vi "1_ImClass(Train).vi"() -> ()   [LabVIEW 2020]
doc: "This example demonstrates the usage of Deep Learning Toolkit for solving hand written digit recognition problem with Convolutional Neural Network (CNN).\n\nDataset: MNIST http://yann.lecun.com/exdb/mnist/\nRequirements: Deep Learning Toolkit for LabVIEW."
uses:
  <vilib>/Ngene/Deep Learning Toolkit/Toolkit/NN_Train/Controls/NN_Train_Params.ctl
  <vilib>/Ngene/Deep Learning Toolkit/Toolkit/NN_Train/Controls/NN_Train_Optimizer.ctl
  <vilib>/Ngene/Deep Learning Toolkit/Toolkit/NN_Train/Controls/NN_Train_Data_Sampling.ctl
  Controls/Img_RGB.ctl
  <vilib>/Ngene/Deep Learning Toolkit/Toolkit/NN_Train/Controls/NN_Train_Session_Data.ctl
  <vilib>/Ngene/Deep Learning Toolkit/Toolkit/NN_Train/Controls/NN_LR_Policy_Cfg.ctl
  <vilib>/Ngene/Deep Learning Toolkit/Toolkit/NN_Train/Controls/NN_LR_Policy_Type.ctl
  <vilib>/Ngene/Deep Learning Toolkit/Toolkit/NN_Network/Controls/NN_Device.ctl
  <vilib>/Ngene/Deep Learning Toolkit/Toolkit/NN_Layers/Layers/FC/Controls/NN_Layer_Config(FC).ctl
  <vilib>/Ngene/Deep Learning Toolkit/Toolkit/NN_Layers/Layers/BatchNorm/Controls/NN_BN_Params.ctl
  <vilib>/Ngene/Deep Learning Toolkit/Toolkit/NN_Activations/Controls/NN_Activation_Type.ctl
  <vilib>/Ngene/Deep Learning Toolkit/Toolkit/NN_Layers/Controls/NN_Layer_Init_Params.ctl
  <vilib>/Ngene/Deep Learning Toolkit/Toolkit/NN_Layers/Controls/NN_Layer_Weight_Init_Type.ctl
  <vilib>/Ngene/Deep Learning Toolkit/Toolkit/NN_Layers/Layers/Input/Controls/NN_Layer_Config(Input3D).ctl
  <vilib>/Ngene/Deep Learning Toolkit/Toolkit/NN_Data/API/NN_Dims(C,H,W).ctl
  <vilib>/Ngene/Deep Learning Toolkit/Toolkit/NN_Data/Controls/NN_Data_type.ctl
  <vilib>/Ngene/Deep Learning Toolkit/Toolkit/NN_Network/Controls/NN_Save_Before_Destroy_Options.ctl
  <vilib>/Ngene/Deep Learning Toolkit/Toolkit/NN_Layers/Layers/Input/Controls/NN_Layer_Config_Aug(Input3D).ctl
  <vilib>/Ngene/Deep Learning Toolkit/Toolkit/NN_Layers/Layers/Input/Controls/Aug/NN_Input3D_Aug_Config.ctl
  <vilib>/Ngene/Deep Learning Toolkit/Toolkit/NN_Layers/Layers/Input/Controls/Aug/NN_Input3D_Aug_Types.ctl
  <vilib>/Ngene/Deep Learning Toolkit/Toolkit/NN_Layers/Layers/Input/Controls/Aug/Aug_Distribution_Type.ctl
  <vilib>/Ngene/Deep Learning Toolkit/Toolkit/NN_Layers/Layers/Input/NN_Layer_Create(Input3D).vi
  <vilib>/Ngene/Deep Learning Toolkit/Toolkit/NN_Layers/Layers/FC/NN_Layer_Create(FC).vi
  <vilib>/Ngene/Deep Learning Toolkit/Toolkit/NN_Layers/Layers/SoftMax/NN_Layer_Create(SoftMax).vi
  <vilib>/Ngene/Deep Learning Toolkit/Toolkit/NN_Train/Loss_Functions/NN_Set_Loss(CrossEntropy).vi
  <vilib>/Ngene/Deep Learning Toolkit/Toolkit/NN_Network/subVIs/NN_Predict/NN_Predict(In3D_Out1D).vi
  <vilib>/Ngene/Deep Learning Toolkit/Toolkit/NN_Train/Eval_Loss/NN_Eval_Test_Error_Loss/NN_Eval(In3D_Out1D).vi
  <vilib>/Ngene/Deep Learning Toolkit/Toolkit/NN_Train/Eval_Loss/NN_Calc_Cofusion_Matrix/NN_Calc_Confusion_Matrix(In3D_Out1D).vi
  <vilib>/Ngene/Deep Learning Toolkit/Toolkit/NN_Data/subVIs/Dataset_Destroy/NN_Datasets_All_Destroy(In3D_Out1D).vi
  <vilib>/Ngene/Deep Learning Toolkit/Toolkit/Deep_Learning_Toolkit_by_Ngene.lvlib
  <vilib>/ptbypt/NI_PtbyPt.lvlib
panel:
  in  "Tab":T1(tab)
  out "Train/Val_Metrics":T2={"Train_Loss"=0.32149845391511916, "Test_Loss"=0.4582325220108032, "Test_Error"=0.14990000426769257} {"Test_Error" format="%#_4g"; "Test_Loss" format="%#_4g"; "Train_Loss" format="%#_4g"}
  in  "Test Images":path=path "D:/DNN/CIFAR-10_Images/Test"
  out "Train Speed (s/iter)":dbl=2166.5318226281724 format="%#_3p"
  out "Train Graphs":T3(graph)={"mean"=0.32149845391511916, "Valid_Loss"=0.45823252, "Valid_Error"=0.1499}
  in  "Eval Test":bool
  out "Session Data":T4={"Epochs"=22.9248, "Tot_Iter"=8955, "LR"=1.25e-05, "LR_iter"=8956}
  in  "Stop":bool
  in  "LR Update Policy":T5={"Policy_Type"=enum."Step", "LR0"=0.0002, "k"=5.0, "WarmUp_Policy"=enum."Step", "WarmUp_Iter"=100, "WarmUp_Ratio"=100.0} {"WarmUp_Ratio" min=1; "WarmUp_Iter" min=1; "LR0" format="%.7f"}
  out "Train Speed (s/iter)":dbl=0.05908060000001569 format="%#_2p"
  in  "Train_Params":T7={"Optimizer"=enum."Adam", "Beta_1"=0.9, "Beta_2"=0.999, "Weight Decay(L1)"=1e-07, "Weight Decay(L2)"=1e-07, "Data_Sampling"=enum."Random"}
  out "Time_Elapsed":dbl=534.0725416999994 format="%<%H:%M:%S>t"
  in  "Working Dir":path=path "D:/working"
  in  "Train Images":path=path "D:/DNN/CIFAR-10_Images/Train"
  in  "NN_Device":T10=enum."GPU"
  out "Incorrectly Classified Imgs":T11[][](array[typedef])=[[{"image"=bytes[30030], "Truth"="airplane", "Predicted"="truck", "Name"="airplane_00003.bmp"}, {"image"=bytes[30030], "Truth"="airplane", "Predicted"="ship", "Name"="airplane_00052.bmp"}, {"image"=bytes[30030], "Truth"="airplane", "Predicted"="bird", "Name"="airplane_00125.bmp"}, {"image"=bytes[30030], "Truth"="airplane", "Predicted"="ship", "Name"="airplane_00169.bmp"}, {"image"=bytes[30030], "Truth"="airplane", "Predicted"="cat", "Name"="airplane_00180.bmp"}, {"image"=bytes[30030], "Truth"="airplane", "Predicted"="truck", "Name"="airplane_00237.bmp"}, {"image"=bytes[30030], "Truth"="airplane", "Predicted"="deer", "Name"="airplane_00255.bmp"}, {"image"=bytes[30030], "Truth"="airplane", "Predicted"="ship", "Name"="airplane_00264.bmp"}, {"image"=bytes[30030], "Truth"="airplane", "Predicted"="automobile", "Name"="airplane_00281.bmp"}, {"image"=bytes[30030], "Truth"="airplane", "Predicted"="truck", "Name"="airplane_00284.bmp"}], [{"image"=bytes[30030], "Truth"="airplane", "Predicted"="ship", "Name"="airplane_00287.bmp"}, {"image"=bytes[30030], "Truth"="airplane", "Predicted"="bird", "Name"="airplane_00313.bmp"}, {"image"=bytes[30030], "Truth"="airplane", "Predicted"="ship", "Name"="airplane_00376.bmp"}, {"image"=bytes[30030], "Truth"="airplane", "Predicted"="bird", "Name"="airplane_00378.bmp"}, {"image"=bytes[30030], "Truth"="airplane", "Predicted"="truck", "Name"="airplane_00398.bmp"}, {"image"=bytes[30030], "Truth"="airplane", "Predicted"="frog", "Name"="airplane_00428.bmp"}, {"image"=bytes[30030], "Truth"="airplane", "Predicted"="truck", "Name"="airplane_00473.bmp"}, {"image"=bytes[30030], "Truth"="airplane", "Predicted"="ship", "Name"="airplane_00477.bmp"}, {"image"=bytes[30030], "Truth"="airplane", "Predicted"="bird", "Name"="airplane_00491.bmp"}, {"image"=bytes[30030], "Truth"="airplane", "Predicted"="ship", "Name"="airplane_00526.bmp"}], [{"image"=bytes[30030], "Truth"="airplane", "Predicted"="cat", "Name"="airplane_00531.bmp"}, {"image"=bytes[30030], "Truth"="airplane", "Predicted"="ship", "Name"="airplane_00581.bmp"}, {"image"=bytes[30030], "Truth"="airplane", "Predicted"="automobile", "Name"="airplane_00675.bmp"}, {"image"=bytes[30030], "Truth"="airplane", "Predicted"="bird", "Name"="airplane_00678.bmp"}, {"image"=bytes[30030], "Truth"="airplane", "Predicted"="cat", "Name"="airplane_00689.bmp"}, {"image"=bytes[30030], "Truth"="airplane", "Predicted"="truck", "Name"="airplane_00767.bmp"}, {"image"=bytes[30030], "Truth"="airplane", "Predicted"="automobile", "Name"="airplane_00814.bmp"}, {"image"=bytes[30030], "Truth"="airplane", "Predicted"="truck", "Name"="airplane_00822.bmp"}, {"image"=bytes[30030], "Truth"="airplane", "Predicted"="ship", "Name"="airplane_00841.bmp"}, {"image"=bytes[30030], "Truth"="airplane", "Predicted"="ship", "Name"="airplane_00885.bmp"}], [{"image"=bytes[30030], "Truth"="airplane", "Predicted"="truck", "Name"="airplane_00886.bmp"}, {"image"=bytes[30030], "Truth"="airplane", "Predicted"="ship", "Name"="airplane_00888.bmp"}, {"image"=bytes[30030], "Truth"="airplane", "Predicted"="cat", "Name"="airplane_00912.bmp"}, {"image"=bytes[30030], "Truth"="airplane", "Predicted"="dog", "Name"="airplane_00982.bmp"}, {"image"=bytes[30030], "Truth"="airplane", "Predicted"="ship", "Name"="airplane_01001.bmp"}, {"image"=bytes[30030], "Truth"="airplane", "Predicted"="automobile", "Name"="airplane_01072.bmp"}, {"image"=bytes[30030], "Truth"="airplane", "Predicted"="ship", "Name"="airplane_01090.bmp"}, {"image"=bytes[30030], "Truth"="airplane", "Predicted"="ship", "Name"="airplane_01093.bmp"}, {"image"=bytes[30030], "Truth"="airplane", "Predicted"="automobile", "Name"="airplane_01109.bmp"}, {"image"=bytes[30030], "Truth"="airplane", "Predicted"="ship", "Name"="airplane_01137.bmp"}], [{"image"=bytes[30030], "Truth"="airplane", "Predicted"="truck", "Name"="airplane_01241.bmp"}, {"image"=bytes[30030], "Truth"="airplane", "Predicted"="truck", "Name"="airplane_01322.bmp"}, {"image"=bytes[30030], "Truth"="airplane", "Predicted"="truck", "Name"="airplane_01461.bmp"}, {"image"=bytes[30030], "Truth"="airplane", "Predicted"="ship", "Name"="airplane_01463.bmp"}, {"image"=bytes[30030], "Truth"="airplane", "Predicted"="truck", "Name"="airplane_01514.bmp"}, {"image"=bytes[30030], "Truth"="airplane", "Predicted"="ship", "Name"="airplane_01574.bmp"}, {"image"=bytes[30030], "Truth"="airplane", "Predicted"="bird", "Name"="airplane_01714.bmp"}, {"image"=bytes[30030], "Truth"="airplane", "Predicted"="ship", "Name"="airplane_01718.bmp"}, {"image"=bytes[30030], "Truth"="airplane", "Predicted"="ship", "Name"="airplane_01739.bmp"}, {"image"=bytes[30030], "Truth"="airplane", "Predicted"="bird", "Name"="airplane_01785.bmp"}], [{"image"=bytes[30030], "Truth"="airplane", "Predicted"="ship", "Name"="airplane_01796.bmp"}, {"image"=bytes[30030], "Truth"="airplane", "Predicted"="horse", "Name"="airplane_01823.bmp"}, {"image"=bytes[30030], "Truth"="airplane", "Predicted"="cat", "Name"="airplane_01898.bmp"}, {"image"=bytes[30030], "Truth"="airplane", "Predicted"="ship", "Name"="airplane_01926.bmp"}, {"image"=bytes[30030], "Truth"="airplane", "Predicted"="automobile", "Name"="airplane_02085.bmp"}, {"image"=bytes[30030], "Truth"="airplane", "Predicted"="bird", "Name"="airplane_02091.bmp"}, {"image"=bytes[30030], "Truth"="airplane", "Predicted"="truck", "Name"="airplane_02136.bmp"}, {"image"=bytes[30030], "Truth"="airplane", "Predicted"="cat", "Name"="airplane_02232.bmp"}, {"image"=bytes[30030], "Truth"="airplane", "Predicted"="ship", "Name"="airplane_02248.bmp"}, {"image"=bytes[30030], "Truth"="airplane", "Predicted"="automobile", "Name"="airplane_02276.bmp"}], [{"image"=bytes[30030], "Truth"="airplane", "Predicted"="bird", "Name"="airplane_02322.bmp"}, {"image"=bytes[30030], "Truth"="airplane", "Predicted"="ship", "Name"="airplane_02379.bmp"}, {"image"=bytes[30030], "Truth"="airplane", "Predicted"="deer", "Name"="airplane_02404.bmp"}, {"image"=bytes[30030], "Truth"="airplane", "Predicted"="ship", "Name"="airplane_02473.bmp"}, {"image"=bytes[30030], "Truth"="airplane", "Predicted"="automobile", "Name"="airplane_02490.bmp"}, {"image"=bytes[30030], "Truth"="airplane", "Predicted"="automobile", "Name"="airplane_02532.bmp"}, {"image"=bytes[30030], "Truth"="airplane", "Predicted"="bird", "Name"="airplane_02548.bmp"}, {"image"=bytes[30030], "Truth"="airplane", "Predicted"="truck", "Name"="airplane_02587.bmp"}, {"image"=bytes[30030], "Truth"="airplane", "Predicted"="bird", "Name"="airplane_02622.bmp"}, {"image"=bytes[30030], "Truth"="airplane", "Predicted"="ship", "Name"="airplane_02672.bmp"}], [{"image"=bytes[30030], "Truth"="airplane", "Predicted"="ship", "Name"="airplane_02704.bmp"}, {"image"=bytes[30030], "Truth"="airplane", "Predicted"="automobile", "Name"="airplane_02782.bmp"}, {"image"=bytes[30030], "Truth"="airplane", "Predicted"="ship", "Name"="airplane_02958.bmp"}, {"image"=bytes[30030], "Truth"="airplane", "Predicted"="bird", "Name"="airplane_02968.bmp"}, {"image"=bytes[30030], "Truth"="airplane", "Predicted"="truck", "Name"="airplane_02976.bmp"}, {"image"=bytes[30030], "Truth"="airplane", "Predicted"="cat", "Name"="airplane_03097.bmp"}, {"image"=bytes[30030], "Truth"="airplane", "Predicted"="bird", "Name"="airplane_03100.bmp"}, {"image"=bytes[30030], "Truth"="airplane", "Predicted"="ship", "Name"="airplane_03158.bmp"}, {"image"=bytes[30030], "Truth"="airplane", "Predicted"="bird", "Name"="airplane_03164.bmp"}, {"image"=bytes[30030], "Truth"="airplane", "Predicted"="automobile", "Name"="airplane_03171.bmp"}]]
  out "Confusion Matrix":string[][](table)=[["771", "28", "44", "15", "13", "3", "5", "5", "71", "45", "0.7710"], ["6", "928", "0", "2", "3", "1", "1", "1", "10", "48", "0.9280"], ["35", "4", "727", "51", "62", "48", "34", "12", "21", "6", "0.7270"], ["15", "6", "46", "665", "29", "149", "33", "16", "22", "19", "0.6650"], ["2", "1", "47", "57", "800", "35", "12", "32", "12", "2", "0.8000"], ["2", "1", "32", "134", "13", "768", "12", "22", "6", "10", "0.7680"], ["5", "4", "42", "66", "34", "15", "822", "3", "6", "3", "0.8220"], ["5", "1", "15", "64", "51", "67", "4", "781", "2", "10", "0.7810"], ["33", "23", "3", "3", "2", "1", "1", "0", "905", "29", "0.9050"], ["4", "37", "4", "4", "1", "2", "2", "1", "16", "929", "0.9290"], ["0.8781", "0.8984", "0.7573", "0.6268", "0.7937", "0.7052", "0.8877", "0.8946", "0.8450", "0.8438", ""]]
  out "Test_Error(Final)":sgl=0.1904
  out "Test_Loss(Final)":sgl=0.544509 format="%#_3g"
  out "Test_Error":sgl=0.1945
  out "Test_Loss":sgl=0.57450217
  # "6. Periodically press \"Eval Test\" button to evaluate Test Loss/Error.\n7. Hit the \"Stop\" button when the Test loss/errors stops decreasing.\n8. Go to the \"Incorrectly Classified Images\" tab to view images from the test dataset that were incorrectly classified.\n9. Navigate to the \"Confusion Matrix\" tab to analyze the classification performance across all classes.\n10. Check the files generated in the \"Working Dir\" directory. A subdirectory with the network name will be created, containing three files: the model configuration file (.cfg), trained weights file (.bin), and a network visualization file (.svg) that can be opened in a web browser.\n\nMore Examples:  https://github.com/ngenehub/deepltk_examples"
  # "Overview: This example demonstrates the usage of Deep Learning Toolkit for solving image classification problem.\nRequirements: \nDeep Learning Toolkit for LabVIEW.\nNI Vision Development Module.\nInstructions:\n1. Provide the train and test dataset paths in the \"Train Images\" and \"Test Images\" control .\n2. Set appropriate path at \"Working Dir\" control where the results of the training will be stored.\n3. Select CPU or GPU at \"NN_Device\" depending on GPU availability.\n4. Run the VI with current configuration of the training parameters and Learning Rate update policy.\n5. Observe how the training loss is decreasing."
  # "Displaying images from the dataset that were incorrectly classified by the trained network."
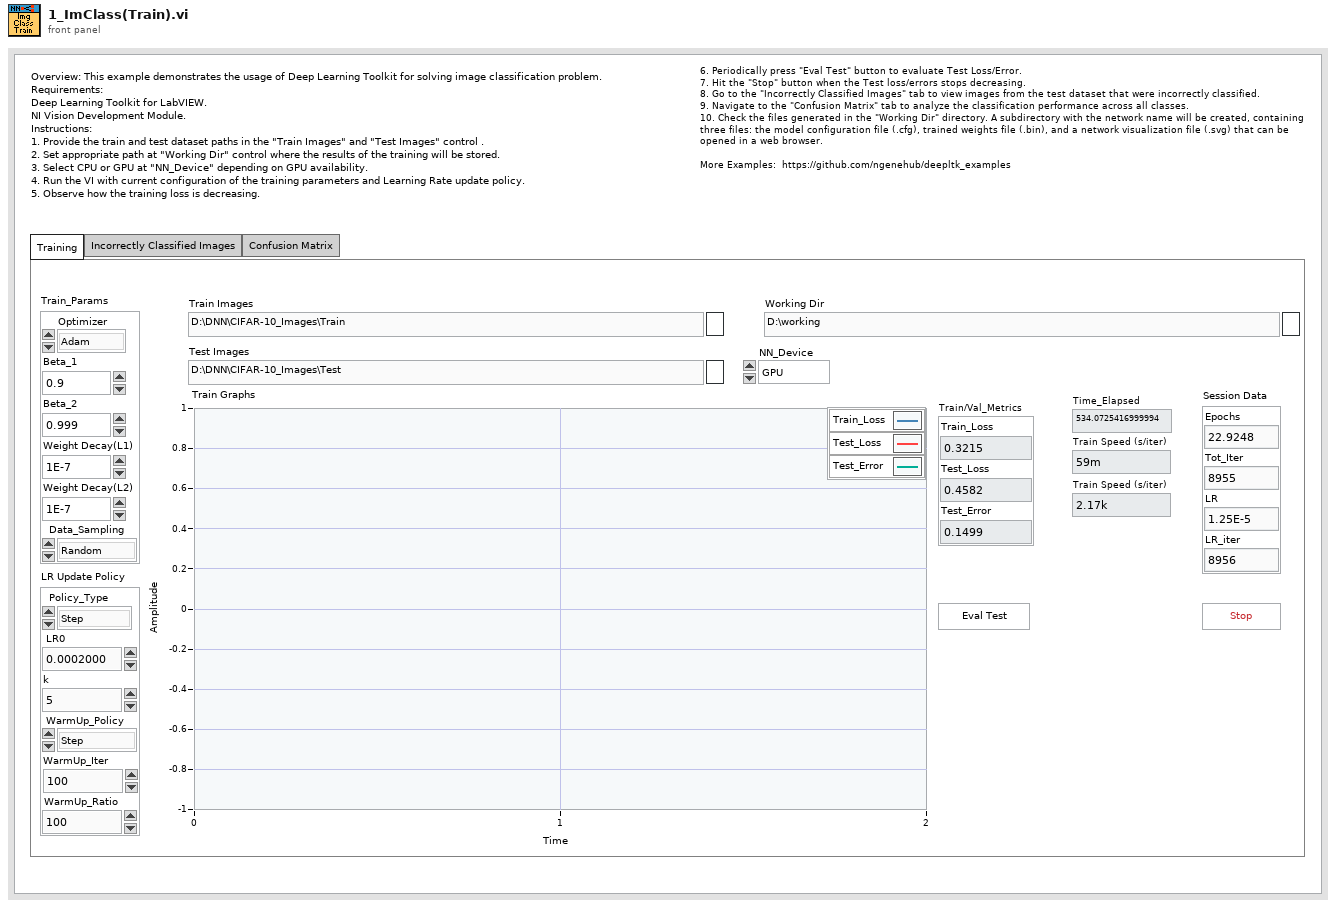
[diagram p1: front panel]
types:
  T1 = enum32{"Training", "Incorrectly Classified Images", "Confusion Matrix"}
  T2 = cluster{"Train_Loss":dbl, "Test_Loss":dbl, "Test_Error":dbl}
  T3 = cluster{"mean":dbl, "Valid_Loss":sgl, "Valid_Error":sgl}
  T4 = typedef "Deep_Learning_Toolkit_by_Ngene.lvlib/NN_Train_Session_Data.ctl" = cluster{"Epochs":sgl, "Tot_Iter":i32, "LR":sgl, "LR_iter":i32}
  T5 = typedef "Deep_Learning_Toolkit_by_Ngene.lvlib/NN_LR_Policy_Cfg.ctl" = cluster{"Policy_Type":T6, "LR0":dbl, "k":sgl, "WarmUp_Policy":enum16{"Step", "Ramp"}, "WarmUp_Iter":i32, "WarmUp_Ratio":sgl}
  T6 = typedef "Deep_Learning_Toolkit_by_Ngene.lvlib/NN_LR_Policy_Type.ctl" = enum16{"Manual", "Step", "Exp", "1/t"}
  T7 = typedef "Deep_Learning_Toolkit_by_Ngene.lvlib/NN_Train_Params.ctl" = cluster{"Optimizer":T8, "Beta_1":sgl, "Beta_2":sgl, "Weight Decay(L1)":sgl, "Weight Decay(L2)":sgl, "Data_Sampling":T9}
  T8 = typedef "Deep_Learning_Toolkit_by_Ngene.lvlib/NN_Train_Optimizer.ctl" = enum16{"SGD", "Adam", "Adagrad", "Adadelta", "RMSProp", "Nesterov"}
  T9 = typedef "Deep_Learning_Toolkit_by_Ngene.lvlib/NN_Train_Data_Sampling.ctl" = enum16{"Random", "Sequential"}
  T10 = typedef "Deep_Learning_Toolkit_by_Ngene.lvlib/NN_Device.ctl" = enum16{"CPU", "GPU"}
  T11 = typedef "Img_RGB.ctl" = cluster{"image":picture, "Truth":string, "Predicted":string, "Name":string}
  T12 = typedef "Deep_Learning_Toolkit_by_Ngene.lvlib/NN_Dims(C,H,W).ctl" = cluster{"C":i32, "H":i32, "W":i32}
  T13 = typedef "Deep_Learning_Toolkit_by_Ngene.lvlib/NN_Layer_Config_Aug(Input3D).ctl" = T14[]
  T14 = typedef "Deep_Learning_Toolkit_by_Ngene.lvlib/NN_Input3D_Aug_Config.ctl" = cluster{"Aug Type":T15, "Aug Value":sgl, "Distribution Type":T16}
  T15 = typedef "Deep_Learning_Toolkit_by_Ngene.lvlib/NN_Input3D_Aug_Types.ctl" = enum16{"Flip_H", "Flip_V", "Brightness", "Contrast", "Noise", "Blur", "Saturation", "Rotate", "Move", "Skew_X", "Skew_Y", "Zoom"}
  T16 = typedef "Deep_Learning_Toolkit_by_Ngene.lvlib/Aug_Distribution_Type.ctl" = enum16{"Uniform", "Gaussian"}
  T17 = typedef "Deep_Learning_Toolkit_by_Ngene.lvlib/NN_Save_Before_Destroy_Options.ctl" = cluster{"CFG?":bool, "Weights?":bool, "Render?":bool}
  T18 = typedef "Deep_Learning_Toolkit_by_Ngene.lvlib/NN_Layer_Config(Input3D).ctl" = cluster{"Name":string, "Dims":T12, "Data_Type":T19, "Shifts":sgl[], "Scales":sgl[]}
  T19 = typedef "Deep_Learning_Toolkit_by_Ngene.lvlib/NN_Data_type.ctl" = enum16{"I8", "U8", "I16", "U16", "U32 ARGB", "SGL"}
  T20 = typedef "Deep_Learning_Toolkit_by_Ngene.lvlib/NN_Layer_Config(FC).ctl" = cluster{"Name":string, "Size":i32, "BN":bool, "BN_Params":T21, "Activation":T22, "Has Bias?":bool, "Init_Params":T23, "Custom_Params":string}
  T21 = typedef "Deep_Learning_Toolkit_by_Ngene.lvlib/NN_BN_Params.ctl" = cluster{"epsilon":sgl, "momentum":sgl}
  T22 = typedef "Deep_Learning_Toolkit_by_Ngene.lvlib/NN_Activation_Type.ctl" = enum16{"Sigmoid", "ReLU", "LReLU", "ReLU6", "GELU", "tanh", "Swish", "Mish", "None"}
  T23 = typedef "Deep_Learning_Toolkit_by_Ngene.lvlib/NN_Layer_Init_Params.ctl" = cluster{"Init_Type":T24, "Value":sgl}
  T24 = typedef "Deep_Learning_Toolkit_by_Ngene.lvlib/NN_Layer_Weight_Init_Type.ctl" = enum16{"Const", "Uniform", "Gaussian", "Xavier"}
  T25 = typedef "Deep_Learning_Toolkit_by_Ngene.lvlib/NN_DataSets_All(In3D_Out1D).ctl" = cluster{"Train":T26, "Validation":T26, "Test":T26}
  T26 = typedef "Deep_Learning_Toolkit_by_Ngene.lvlib/NN_DataSet(In3D_Out1D).ctl" = cluster{"Inputs Ref.":variant, "Outputs Ref.":T27, "Dataset_Size":i32, "Dims_In":T12, "Dims_Out":i32, "Labels":string[], "File Paths":path[], "Custom_Data":variant}
  T27 = typedef "Deep_Learning_Toolkit_by_Ngene.lvlib/NN_Data_ref(2D_SGL).ctl" = refnum<data-value>
  T28 = typedef "Deep_Learning_Toolkit_by_Ngene.lvlib/NN.ctl" = cluster{"Name":string, "No of Layers":i32, "mBatch":i32, "Layers":T29[], "Dimty":T30, "Dims_In":T12, "Dims_Out":T12, "Working_Dir":path, "Train?":bool, "Train_Params":T7, "LR_Update_Policy":T5, "Session Data":T4, "Ground_truth":T31, "NNg_hdls":T32, "NN_Device":T10, "GPU Id":i32, "Labels":string[], "Loss_Type":T33, "Loss_Cfg_Prms":variant, "NNG_WS":T34, "DryRun?":bool}
  T29 = typedef "Deep_Learning_Toolkit_by_Ngene.lvlib/NN_Layer_ref.ctl" = refnum<file>
  T30 = typedef "Deep_Learning_Toolkit_by_Ngene.lvlib/NN_In_Out_Dim-ty.ctl" = enum8{"In1D_Out1D", "In3D_Out1D", "In3D_Out3D", "In3D_OutBBox"}
  T31 = typedef "Deep_Learning_Toolkit_by_Ngene.lvlib/NN_Ground_truth.ctl" = cluster{"Y":variant}
  T32 = typedef "Deep_Learning_Toolkit_by_Ngene.lvlib/nng_cuda_handles.ctl" = cluster{"cudnn":u64, "cublas":u64, "stream":u64, "curand":u64}
  T33 = typedef "Deep_Learning_Toolkit_by_Ngene.lvlib/NN_Loss_Type.ctl" = enum16{"None", "MSE", "CrossEntropy", "YOLO_v2", "YOLO_v4"}
  T34 = typedef "Deep_Learning_Toolkit_by_Ngene.lvlib/NNG_WS.ctl" = cluster{"NNG_WS_Mem":T35, "Max_WS_Size":i64}
  T35 = typedef "Deep_Learning_Toolkit_by_Ngene.lvlib/NNg_WS_Mem_DVR.ctl" = refnum<data-value>
  T36 = typedef "Deep_Learning_Toolkit_by_Ngene.lvlib/NN_Eval_Params.ctl" = cluster{"Loss":sgl, "Error":sgl}
  T37 = cluster{"mean":dbl, "Test_Loss":sgl, "Test_Error":sgl}
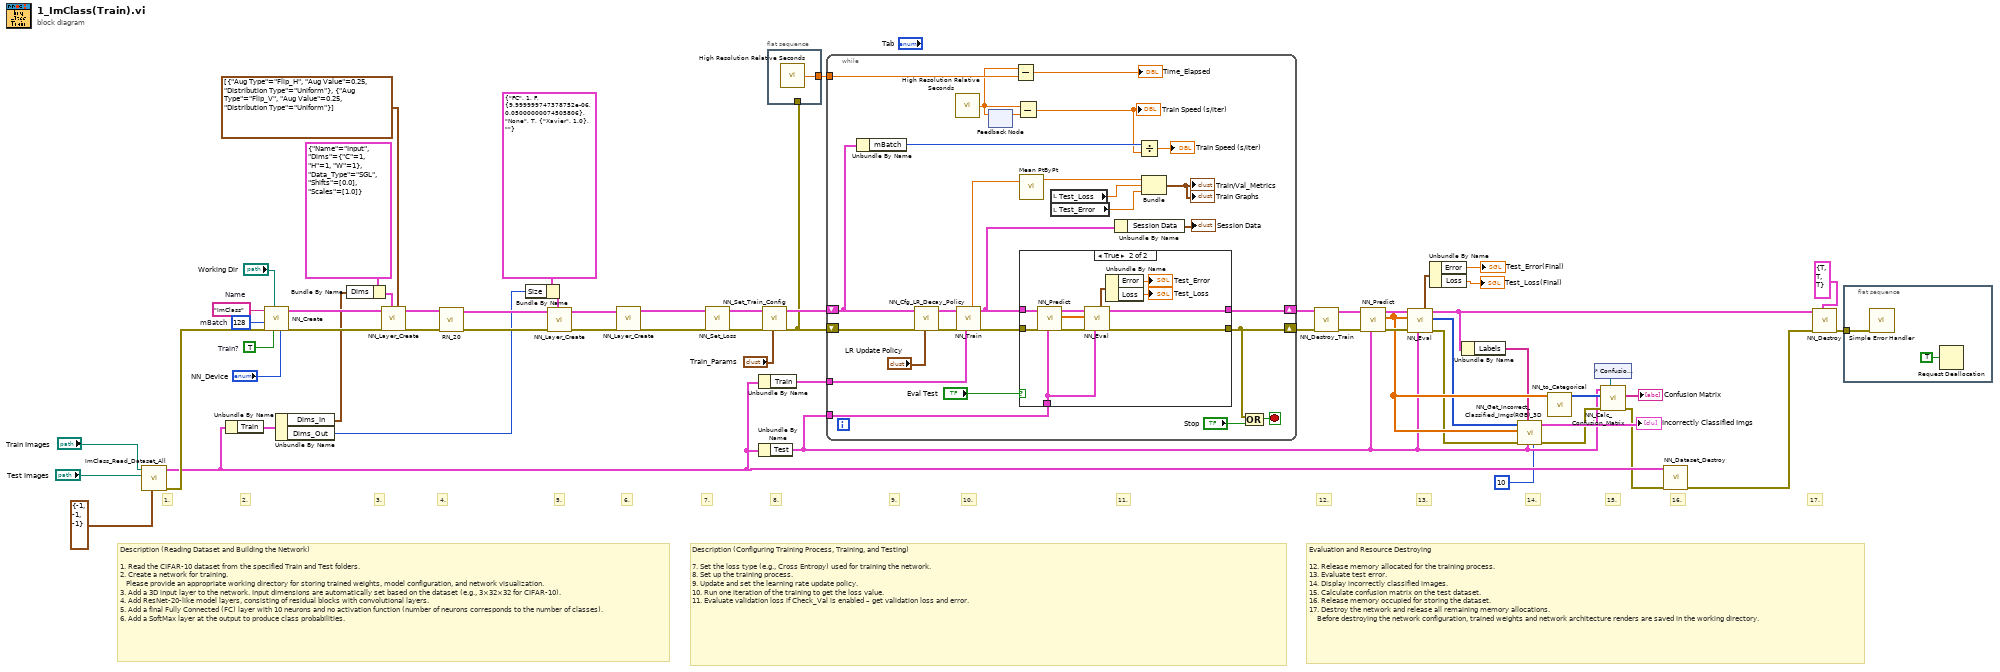
[diagram p0: block diagram]
diagram:
  w44 = TRUE  # Train?
  w53 = 128  # mBatch
  w59 = "ImClass"  # Name
  # "Evaluation and Resource Destroying\n\n12. Release memory allocated for the training process.\n13. Evaluate test error.\n14. Display incorrectly classified images.\n15. Calculate confusion matrix on the test dataset.\n16. Release memory occupied for storing the dataset.\n17. Destroy the network and release all remaining memory allocations.\n    Before destroying the network configuration, trained weights and network architecture renders are saved in the working directory."
  # "Description (Configuring Training Process, Training, and Testing)\n\n7. Set the loss type (e.g., Cross Entropy) used for training the network.\n8. Set up the training process.\n9. Update and set the learning rate update policy.\n10. Run one iteration of the training to get the loss value.\n11. Evaluate validation loss if Check_Val is enabled – get validation loss and error."
  # "Description (Reading Dataset and Building the Network)\n\n1. Read the CIFAR-10 dataset from the specified Train and Test folders.\n2. Create a network for training.\n   Please provide an appropriate working directory for storing trained weights, model configuration, and network visualization.\n3. Add a 3D input layer to the network. Input dimensions are automatically set based on the dataset (e.g., 3×32×32 for CIFAR-10).\n4. Add ResNet-20-like model layers, consisting of residual blocks with convolutional layers.\n5. Add a final Fully Connected (FC) layer with 10 neurons and no activation function (number of neurons corresponds to the number of classes).\n6. Add a SoftMax layer at the output to produce class probabilities."
  # "7."
  # "17."
  # "15."
  # "16."
  # "14."
  # "13."
  # "12."
  # "11."
  # "10."
  # "9."
  # "8."
  # "6."
  # "5."
  # "4."
  # "3."
  # "2."
  # "1."
  n1 = call "ImClass_Read_Dataset_All.vi"("Dims(C,H,W)"=T12 {"C"=-1, "H"=-1, "W"=-1}, "Test Path"="Test Images", "Train Path"="Train Images") -> ("error out"=w60:errorcluster, "Dataset"=w30:T25)  [unwired: 7 in]
  n2 = Unbundle By Name(w30) -> ("Train"=w29:T26)
  n3 = call <vilib>:"NN_Create.vi"("NN_Device"="NN_Device", "Train? (false)"=w44, "Working Dir"="Working Dir", "error in (no error)"=w60, "mBatch (1)"=w53, "Name"=w59) -> ("error out"=w57:errorcluster, "NN out"=w58:T28)  [unwired: 4 in]
  n4 = Unbundle By Name(w29) -> ("Dims_In"=w31:T12, "Dims_Out"=w3:i32)
  n5 = Bundle By Name(cluster=T18 {"Name"="Input", "Dims"={"C"=1, "H"=1, "W"=1}, "Data_Type"=enum."SGL", "Shifts"=[0.0], "Scales"=[1.0]} ("Cluster"), "Dims"=w31) -> (w48:T18)
  n6 = call-poly <vilib>:"NN_Layer_Create.vi"("Aug Config Params(3D)"=T13 [{"Aug Type"=enum."Flip_H", "Aug Value"=0.25, "Distribution Type"=enum."Uniform"}, {"Aug Type"=enum."Flip_V", "Aug Value"=0.25, "Distribution Type"=enum."Uniform"}], "Input3D_Cfg"=w48, "error in (no error)"=w57, "NN In"=w58) -> ("error out"=w38:errorcluster, "NN out"=w20:T28)  [unwired: 5 in, 1 out]
  n7 = call "RN_20.vi"("error in (no error)"=w38, "NN in"=w20) -> ("error out"=w40:errorcluster, "NN out"=w39:T28)  [unwired: 8 in]
  n8 = Bundle By Name(cluster=T20 {"Name"="FC", "Size"=1, "BN"=FALSE, "BN_Params"={"epsilon"=1e-05, "momentum"=0.05}, "Activation"=enum."None", "Has Bias?"=TRUE, "Init_Params"={"Init_Type"=enum."Xavier", "Value"=1.0}, "Custom_Params"=""} ("Layer_Config_Params"), "Size"=w3) -> (w37:T20)
  n9 = call-poly <vilib>:"NN_Layer_Create.vi"("FC_Cfg"=w37, "error in (no error)"=w40, "NN in"=w39) -> ("error out"=w51:errorcluster, "NN out"=w52:T28)  [unwired: 6 in, 1 out]
  n10 = call-poly <vilib>:"NN_Layer_Create.vi"("error in (no error)"=w51, "NN in"=w52) -> ("error out"=w34:errorcluster, "NN out"=w36:T28)  [unwired: 7 in, 1 out]
  n11 = call-poly <vilib>:"NN_Set_Loss.vi"("error in (no error)"=w34, "NN in"=w36) -> ("error out"=w33:errorcluster, "NN out"=w35:T28)  [unwired: 8 in]
  n12 = Unbundle By Name(w30) -> ("Train"=w32:T26)
  n13 = Unbundle By Name(w30) -> ("Test"=w4:T26)
  n14 = call <vilib>:"NN_Set_Train_Config.vi"("NN_Train_Params"="Train_Params", "error in (no error)"=w33, "NN in"=w35) -> ("error out"=w45:errorcluster, "NN out"=w46:T28)  [unwired: 7 in]
  n15 = flat-sequence {
    tunnel: [w61] -> w55
    tunnel: w45 -> [_]
    frame #0 {
      n16 = call <vilib>:"High Resolution Relative Seconds.vi"() -> ("relative seconds"=w61:dbl)
    }
  }
  n17 = while {
    shift-right: [w70] -> w25
    shift-left: w45 -> [w64]
    shift-right: [w67] -> w26
    shift-left: w46 -> [w65]
    tunnel: w55 -> [w79]
    tunnel: w32 -> [w69]
    tunnel: w4 -> [w63]
    stop <- w86 stop-if-true
    n18 = Unbundle By Name(w65) -> ("mBatch"=w75:i32)
    n19 = call <vilib>:"NN_Cfg_LR_Decay_Policy.vi"("LR_Decay_Params"="LR Update Policy", "error in (no error)"=w64, "NN in"=w65) -> ("error out"=w81:errorcluster, "NN out"=w87:T28)  [unwired: 7 in]
    n20 = call <vilib>:"High Resolution Relative Seconds.vi"() -> ("relative seconds"=w78:dbl)
    n21 = call <vilib>:"NN_Train.vi"("Train Dataset"=w69, "error in (no error)"=w81, "NN in"=w87) -> ("error out"=w71:errorcluster, "NN out"=w66:T28, "Loss"=w82:sgl)  [unwired: 3 in, 3 out]
    n22 = feedback #1() -> (w88:dbl)  [unwired: 1 in]
    n23 = feedback-in #1(w78) -> ()
    n24 = Subtract(x=w78, y=w79) -> (x-y=→"Time_Elapsed":dbl)
    n25 = Subtract(x=w78, y=w88) -> (x-y=w73:dbl)
    "Train Speed (s/iter)" <- w73
    n26 = call <vilib>:"Mean PtByPt.vi"("x"=w82) -> ("mean"=w83:dbl)  [unwired: 3 in, 1 out]
    n27 = case shown="True" "Eval Test" {
      tunnel: w66 -> [w89 w101]
      tunnel: w71 -> [w90 w97]
      tunnel: [w90 w99] -> w70
      tunnel: [w89 w100] -> w67
      tunnel: w63 -> [_ w94]
      frame False {
      }
      frame True {
        n28 = call-poly <vilib>:"NN_Predict.vi"("Dataset"=w94, "error in (no error)"=w97, "NN in"=w101) -> ("error out"=w96:errorcluster, "Predictions"=w95:sgl[][], "NN out"=w98:T28)  [unwired: 6 in]
        n29 = call-poly <vilib>:"NN_Eval.vi"("Dataset"=w94, "error in (no error)"=w96, "Predictions"=w95, "NN in"=w98) -> ("error out"=w99:errorcluster, "NN out"=w100:T28, "NN_Eval_Params"=w93:T36)  [unwired: 4 in, 1 out]
        n30 = Unbundle By Name(w93) -> ("Error"=→"Test_Error":sgl, "Loss"=→"Test_Loss":sgl)
      }
    }
    n31 = local read "Test_Loss"() -> (w85:sgl)
    n32 = local read "Test_Error"() -> (w80:sgl)
    n33 = Unbundle By Name(w66) -> ("Session Data"=→"Session Data":T4)
    n34 = Divide(x=w75, y=w73) -> (x/y=→"Train Speed (s/iter)":dbl)
    n35 = Bundle("mean"=w83, "Test_Loss"=w85, "Test_Error"=w80) -> (→"Train Graphs" →"Train/Val_Metrics":T37)  [unwired: 1 in]
    n36 = Compound Arithmetic op=OR(w70, "Stop") -> (w86:bool)
  }
  n37 = call <vilib>:"NN_Destroy_Train.vi"("error in (no error)"=w25, "NN in"=w26) -> ("error out"=w22:errorcluster, "NN out"=w24:T28)  [unwired: 8 in]
  n38 = call-poly <vilib>:"NN_Predict.vi"("Dataset"=w4, "error in (no error)"=w22, "NN in"=w24) -> ("error out"=w21:errorcluster, "Predictions"=w18:sgl[][], "NN out"=w23:T28)  [unwired: 6 in]
  n39 = call-poly <vilib>:"NN_Eval.vi"("Dataset"=w4, "error in (no error)"=w21, "Predictions"=w18, "NN in"=w23) -> ("error out"=w17:errorcluster, "Incrct_Class_idx"=w13:i32[], "NN out"=w7:T28, "NN_Eval_Params"=w10:T36)  [unwired: 4 in]
  n40 = Unbundle By Name(w10) -> ("Error"=→"Test_Error(Final)":sgl, "Loss"=→"Test_Loss(Final)":sgl)
  n41 = Unbundle By Name(w7) -> ("Labels"=w6:string[])
  n42 = call "NN_Get_Incorrect_Classified_Imgs(RGB)_3D.vi"("# of columns"=10 ("Report shape"), "Dataset"=w4, "Labels"=w6, "error in (no error)"=w17, "Predictions"=w18, "MisClassed_idx"=w13) -> ("error out"=w16:errorcluster, "Images(GrayScale)"=→"Incorrectly Classified Imgs":T11[][])  [unwired: 4 in]
  n43 = call <vilib>:"NN_to_Categorical.vi"("Prediction"=w18) -> ("Label_Idx"=w19:i32[])  [unwired: 10 in]
  n44 = control-ref of="Confusion Matrix"() -> (w27:refnum<vi>)
  n45 = call-poly <vilib>:"NN_Calc_Confusion_Matrix.vi"("Confusion Matrix (Table) ref."=w27, "error in (no error)"=w16, "Predictions"=w19, "Dataset"=w4) -> ("error out"=w15:errorcluster, "Confusion Matrix (Table)"=→"Confusion Matrix":string[][])  [unwired: 3 in, 3 out]
  n46 = call-poly <vilib>:"NN_Dataset_Destroy.vi"("error in (no error)"=w15, "Datasets_All(In3D_Out1D)"=w30) -> ("error out"=w47:errorcluster)  [unwired: 9 in]
  n47 = call <vilib>:"NN_Destroy.vi"("Save (T, T, T)"=T17 {"CFG?"=TRUE, "Weights?"=TRUE, "Render?"=TRUE} ("Save_Config"), "error in (no error)"=w47, "NN in"=w7) -> ("error out"=w56:errorcluster)  [unwired: 7 in, 1 out]
  n48 = flat-sequence {
    tunnel: w56 -> [w103]
    frame #0 {
      n49 = call <vilib>:"Simple Error Handler.vi"("error in (no error)"=w103) -> ()  [unwired: 4 in, 5 out]
      n50 = Request Deallocation(TRUE ("flag")) -> ()
    }
  }
